vi "Splitters.vi"() -> (4 "Operators":string[](array[string]), 6 "Delimiters":string[](array[string]))   [LabVIEW 2019, in "SLL JSON to Cluster.lvlib"]
doc: "This VI gives operators to classifies input JSON tokens into ints equivalent data type"
uses:
  SLL JSON to Cluster.lvlib
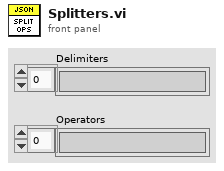
[diagram p1: front panel]
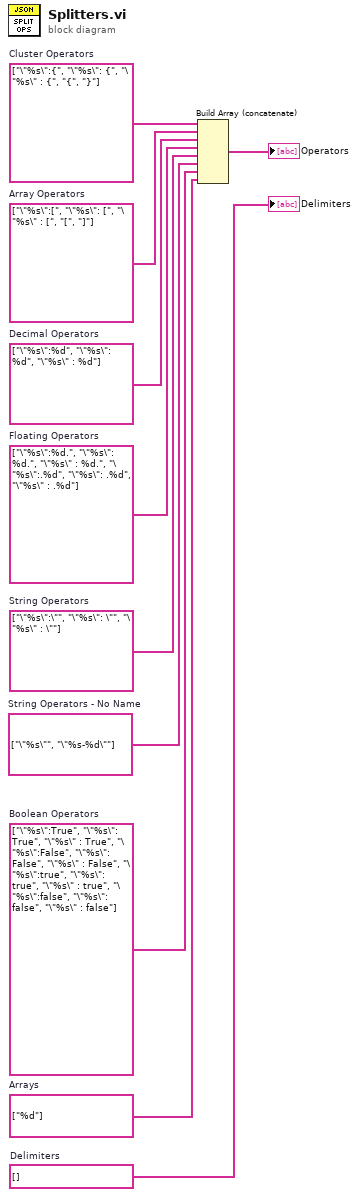
[diagram p0: block diagram]
diagram:
  w10 = string[] ["%d"]  # Arrays
  w9 = string[] ["\"%s\":True", "\"%s\": True", "\"%s\" : True", "\"%s\":False", "\"%s\": False", "\"%s\" : False", "\"%s\":true", "\"%s\": true", "\"%s\" : true", "\"%s\":false", "\"%s\": false", "\"%s\" : false"]  # Boolean Operators
  w7 = string[] ["\"%s\"", "\"%s-%d\""]  # String Operators - No Name
  w6 = string[] ["\"%s\":\"", "\"%s\": \"", "\"%s\" : \""]  # String Operators
  w5 = string[] ["\"%s\":%d.", "\"%s\": %d.", "\"%s\" : %d.", "\"%s\":.%d", "\"%s\": .%d", "\"%s\" : .%d"]  # Floating Operators
  w4 = string[] ["\"%s\":%d", "\"%s\": %d", "\"%s\" : %d"]  # Decimal Operators
  w3 = string[] ["\"%s\":[", "\"%s\": [", "\"%s\" : [", "[", "]"]  # Array Operators
  w2 = string[] ["\"%s\":{", "\"%s\": {", "\"%s\" : {", "{", "}"]  # Cluster Operators
  w1 = string[] []  # Delimiters
  n1 = Build Array (concatenate)(w2, w3, w4, w5, w6, w7, w9, w10) -> (→"Operators":string[])
  "Delimiters" <- w1
